vi "Listener.vi"   [LabVIEW 2013, in "WebSockets.lvlib"]
uses:
  WebSockets.lvlib
  ListenerStates.ctl
  ReadMessage.ctl
types:
  T1 = typedef "WebSockets.lvlib/ReadMessage.ctl" = cluster{"ConnectionID":string, "Data":string}
  T2 = typedef "WebSockets.lvlib/ListenerStates.ctl" = enum16{"Initialise", "Listening", "Exit"}
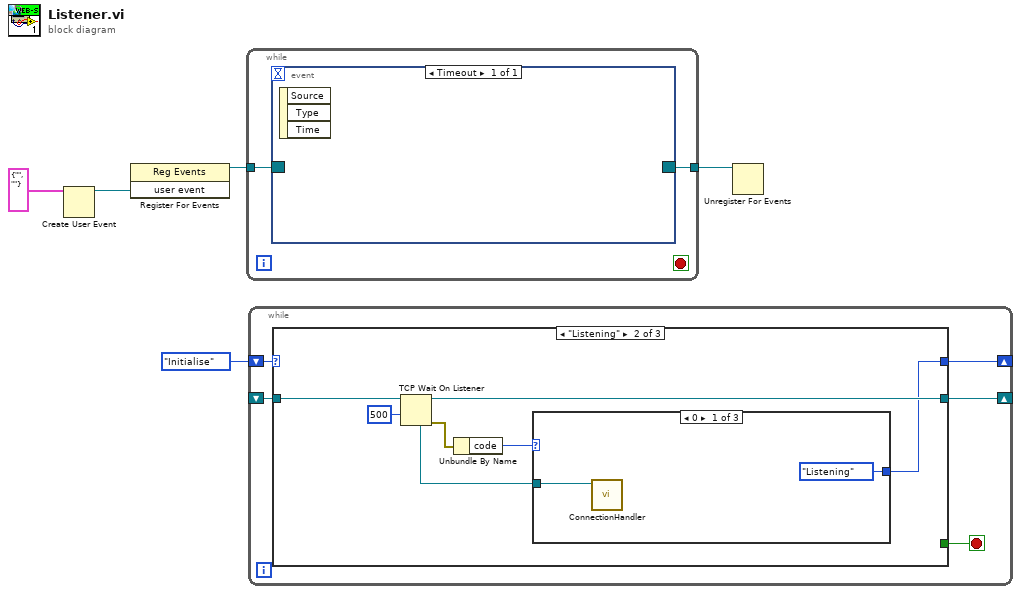
[diagram p0: block diagram]
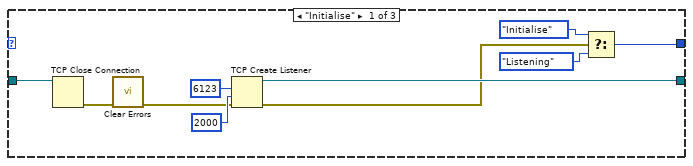
[diagram p2: hidden frame]
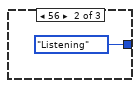
[diagram p3: hidden frame]
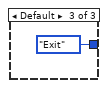
[diagram p4: hidden frame]
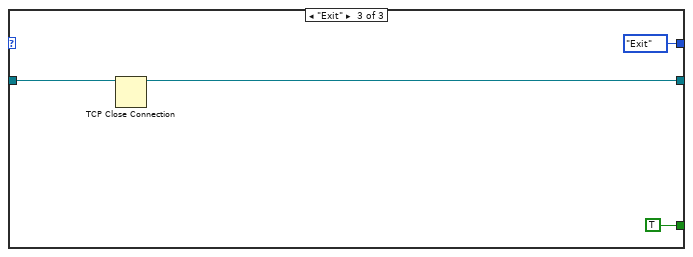
[diagram p5: hidden frame]
diagram:
  n1 = Create User Event(user event datatype=T1 {"ConnectionID"="", "Data"=""}) -> (user event=w4:refnum<user-event>)  [unwired: 1 in, 1 out]
  n2 = register-events(w4) -> (reference out=w3:refnum<event-registration>)  [unwired: 2 in, 1 out]
  n3 = while {
    tunnel: w3 -> [w7]
    tunnel: [w6] -> w2
    stop <- _ stop-if-true
    n4 = event shown="[0] Timeout" {
      selector: w7 -> [_]
      dyn-events: [_] -> w6
      timeout: _ -> [_]
      event Timeout {
        n5 = event-data() -> ()  [unwired: 1 in, 3 out]
      }
    }
  }
  n6 = while {
    shift-right: [w11] -> _
    shift-left: ListenerStates."Initialise" -> [w12]
    shift-right: [w10] -> _
    shift-left: _ -> [w9]
    stop <- w8 stop-if-true
    n7 = case shown="\"Listening\"" w12 {
      tunnel: [w16 w24 ListenerStates."Exit"] -> w11
      tunnel: [w20 w28 w36] -> w10
      tunnel: w9 -> [w15 w29 w37]
      tunnel: [_ _ TRUE] -> w8
      frame "Initialise" {
        n8 = TCP Close Connection(connection ID=w15) -> (error out=w14:errorcluster)  [unwired: 2 in, 1 out]
        n9 = call <vilib>:"Clear Errors.vi"("error in (no error)"=w14) -> ("error out"=w13:errorcluster)  [unwired: 6 in]
        n10 = TCP Create Listener(8:w13, 9:2000 ("timeout ms (25000)"), 10:u16 6123 ("port")) -> (0:w19:errorcluster, 3:w20:refnum<k5>)  [unwired: 2 in, 1 out]
        n11 = Select(t=ListenerStates."Initialise", s=w19, f=ListenerStates."Listening") -> (s? t:f=w16:T2)
      }
      frame "Listening" {
        n12 = TCP Wait On Listener(9:500 ("timeout ms (wait forever: -1)"), 11:w29) -> (0:w26:errorcluster, 3:w28:refnum<k5>, 4:w23:refnum<k5>)  [unwired: 2 in, 2 out]
        n13 = Unbundle By Name(w26) -> ("code"=w25:i32)
        n14 = case shown="0" w25 {
          tunnel: [ListenerStates."Listening" ListenerStates."Listening" ListenerStates."Exit"] -> w24
          tunnel: w23 -> [w30 _ _]
          frame 0 {
            n15 = call "ConnectionHandler.vi"("connection ID"=w30) -> ()  [unwired: 11 in]
          }
          frame 56 {
          }
          frame Default {
          }
        }
      }
      frame "Exit" {
        n16 = TCP Close Connection(connection ID=w37) -> (connection ID out=w36:refnum<k5>)  [unwired: 2 in, 1 out]
      }
    }
  }
  n17 = Unregister For Events(event registration refnum=w2) -> ()  [unwired: 1 in, 1 out]
